vi "F490Y0YIPPPDQXN.vi"() -> ()   [LabVIEW 2014]
uses:
  <vilib>/Utility/error.llb/DialogType.ctl
  <vilib>/addons/Biomedical/Biosignal Measurements/Biosignal Preprocessing/subVIs/bmt_Rate Extractor_peak_valley.ctl
  <vilib>/addons/Biomedical/Biosignal Measurements/Biosignal Preprocessing/Biosignal Rate Extractor (Waveform).vi
  <vilib>/DigilentWF/DigilentWF.lvlib
  <vilib>/addons/Biomedical/NI_BMTK_Measurements.lvlib
panel:
  in  "Acquisition Time":dbl=4.0 caption="Acquisition Time (s) (no change)"
  in  "Sample Rate":dbl=1500.0 caption="Sample Rate (no change)" format="%#_6p"
  in  "On":bool
  in  "UC2":dbl=120.0 caption="Upper Cut-Off"
  in  "LC2":dbl=15.0 caption="Lower Cut-Off"
  out "Smoothing filter":dynamicdata(graph)=[{"t0"=timestamp(0 s since 1904-01-01), "dt"=0.00066667, "Y"=array[6000 elements], "attributes"=variant("NI_ChannelName"=variant(string "Filtered (Filtered)"), "NI_OriginalChannelName"=variant(string "Filtered"))}]
  out "Bandpass filter":dynamicdata(graph)=[{"t0"=timestamp(0 s since 1904-01-01), "dt"=0.00066667, "Y"=array[6000 elements], "attributes"=variant("NI_ChannelName"=variant(string "Filtered (Filtered)"), "NI_OriginalChannelName"=variant(string "Filtered"))}]
  out "Mean Heart Rate":dbl=inf
  in  "HT":dbl(slide)=0.32291666666666663 scale=-0.5..1.5
  in  "LT":dbl(slide)=0.15624999999999997 scale=-0.5..1.5
  out "pulse interval (s)":dbl format="%#.6g"
  out "number of pulses":i32=-1
  out "biosignals":dynamicdata(graph)=[{"t0"=timestamp(0 s since 1904-01-01), "dt"=0.00066667, "Y"=array[6000 elements], "attributes"=variant("NI_ChannelName"=variant(string "Filtered (Filtered)"), "NI_OriginalChannelName"=variant(string "Filtered"))}]
  out "unfiltered":waveform(dbl)(graph)={"t0"=timestamp(3549308991.8308573 s since 1904-01-01), "dt"=0.00066667, "Y"=array[6000 elements]}
  out "Bandpass filter":dynamicdata(graph)=[{"t0"=timestamp(0 s since 1904-01-01), "dt"=0.00066667, "Y"=array[6000 elements], "attributes"=variant("NI_ChannelName"=variant(string "Filtered"))}]
  in  "UC1":dbl=34.0 caption="Upper Cut-Off"
  out "Averaged":waveform(dbl)(graph)={"t0"=timestamp(0 s since 1904-01-01), "dt"=0.00066667, "Y"=array[6000 elements]}
  in  "Samples to Average":i32=10 min=1
  in  "LC1":dbl=1.0 caption="Lower Cut-Off"
  in  "-5V Supply":bool=TRUE
  in  "+5V Supply":bool=TRUE
  in  "Master Enable":bool=TRUE
  in  "V 2":dbl=5.0 caption="Voltage" min=0.5 max=5.0 step=0.1
  in  "V":dbl=-5.0 caption="Voltage" min=-5.0 max=-0.5 step=0.1
  in  "Device Name":string="Analog Discovery 2"
  in  "Stop":bool
  in  "Analog Channel":string="mso/1" caption="Channel"
  # "Heart Rate"
  # "Analog Discovery 2\nPower Supplies"
  # "Analog Discovery MSO Settings"
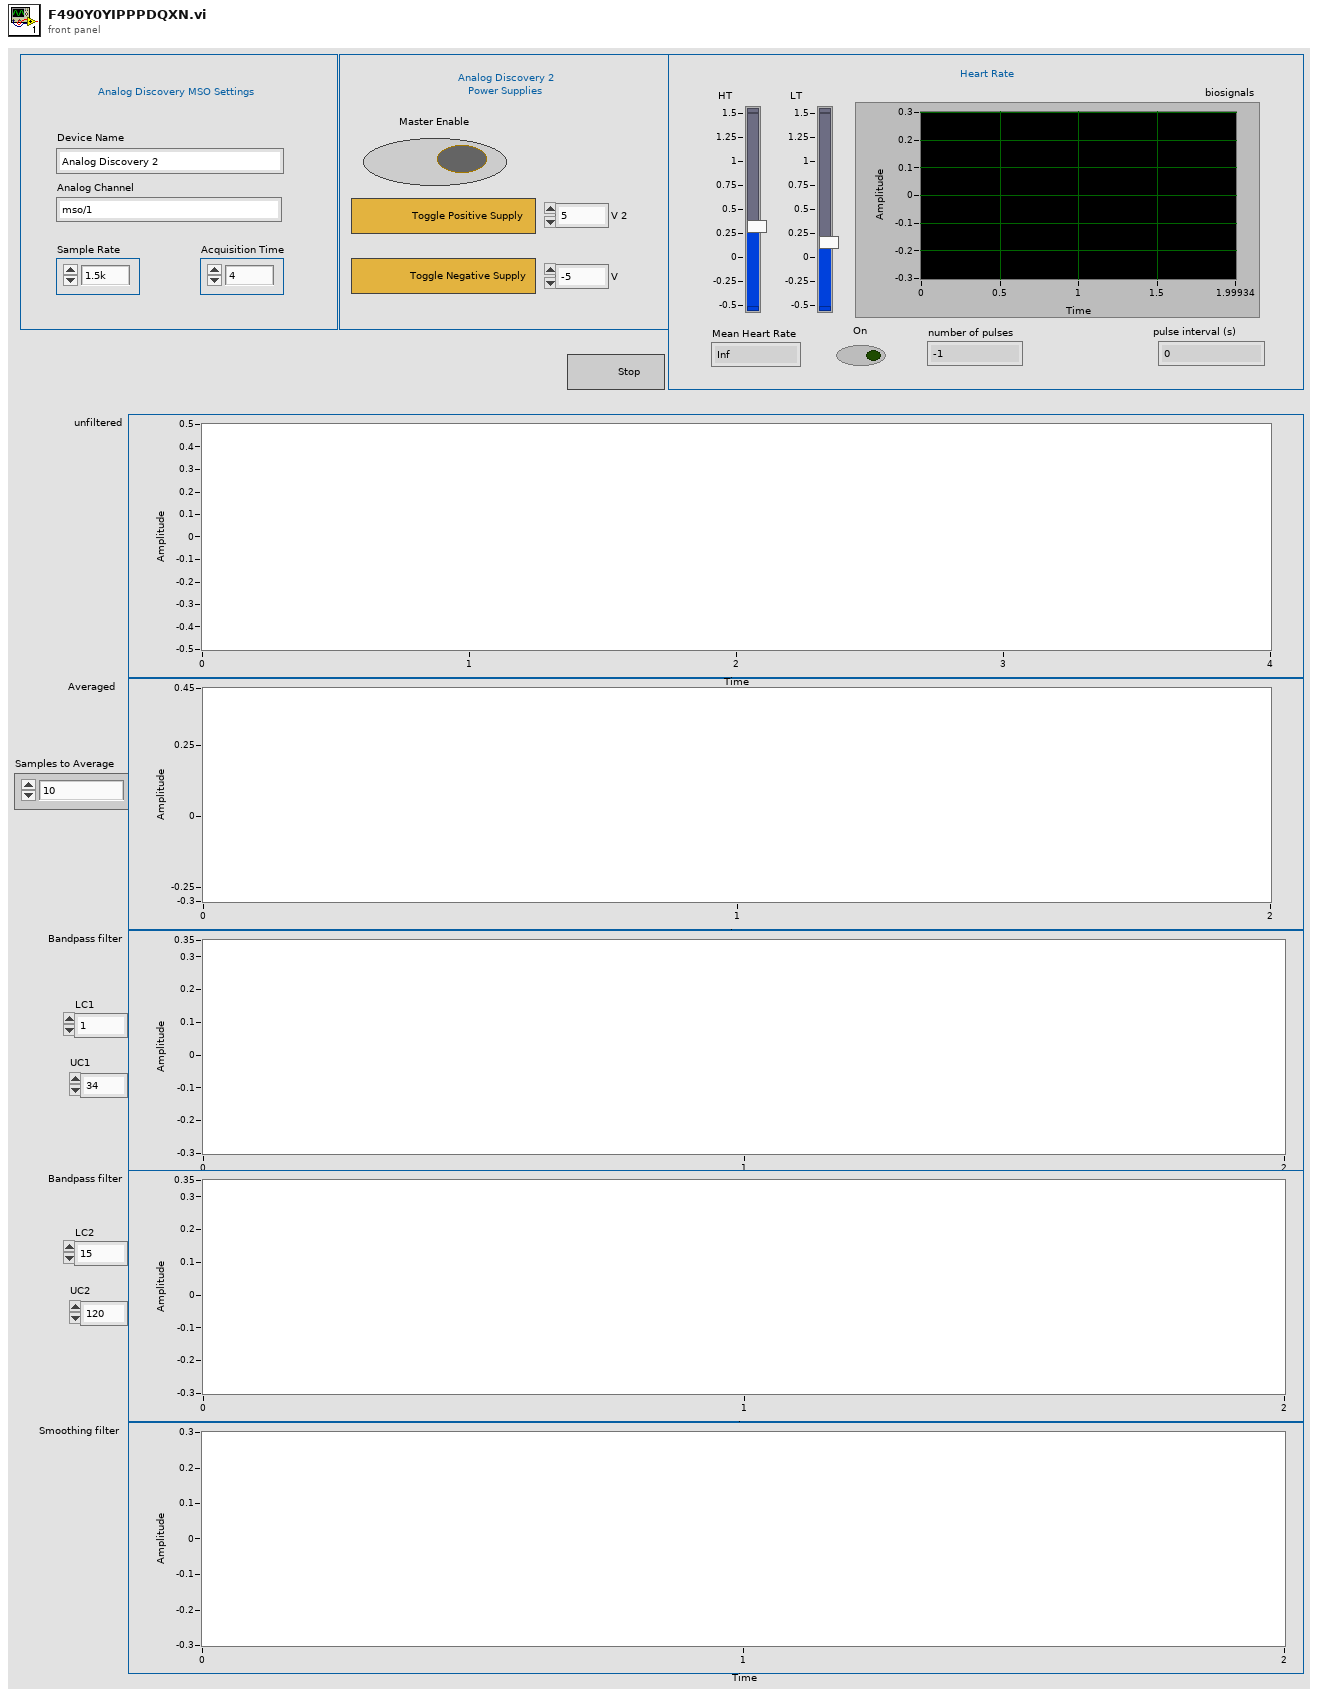
[diagram p1: front panel]
types:
  T1 = typedef "DialogType.ctl" = u16
  T2 = typedef "NI_BMTK_Measurements.lvlib/bmt_Rate Extractor_peak_valley.ctl" = u16
  T3 = typedef "LVCursorListTypeDef.ctl" = cluster{"Name":string, "Color":u32, "Style":u8, "Point Style":u8, "Name Visible":bool, "Allow Drag":bool, "Cursor Mode":u32, "Plot":i32, "Index":i32, "Position":cluster{"X":dbl, "Y":dbl}, "X Scale":u32, "Y Scale":u32, "Watch Plots":i32[], "Watch All Plots":bool, "Plot Area":i32, "Label Offset":cluster{"X":dbl, "Y":dbl}}[]
  T4 = cluster{"Name":string, "Color":u32, "Style":u8, "Point Style":u8, "Name Visible":bool, "Allow Drag":bool, "Cursor Mode":u32, "Plot":i32, "Index":i32, "Position":cluster{"X":dbl, "Y":dbl}, "X Scale":u32, "Y Scale":u32, "Watch Plots":i32[], "Watch All Plots":bool, "Plot Area":i32, "Label Offset":cluster{"X":dbl, "Y":dbl}}
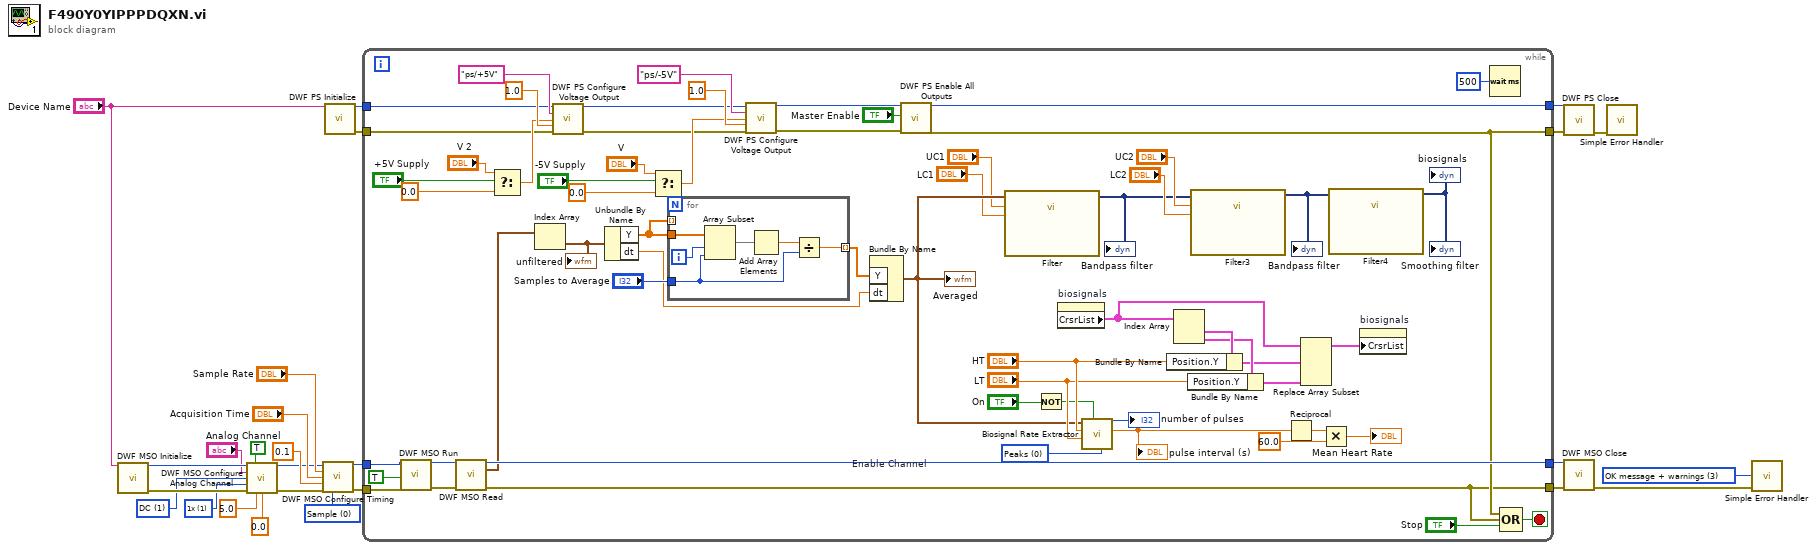
[diagram p0: block diagram]
diagram:
  w6 = 0 items=["Sample", "Peak Detect"] ("Sampling Mode")
  w19 = 1 items=["1x"=1, "10x"=10] ("Probe Attenuation")
  w20 = 1 items=["AC", "DC"] ("Vertical Coupling")
  w25 = TRUE  # Enable Channel
  w26 = T1 3 items=["no dialog", "OK message", "continue or stop message", "OK message + warnings", "continue/stop + warnings"] ("type of dialog (OK msg:1)")
  n1 = call <vilib>:"DWF MSO Initialize.vi"("Device Name"="Device Name") -> ("Instrument Handle Out"=w23:u32, "Error Out"=w24:errorcluster)  [unwired: 13 in]
  n2 = call <vilib>:"DWF MSO Configure Analog Channel.vi"("Instrument Handle In"=w23, "Enable Channel"=w25, "Channel"="Analog Channel", "Vertical Coupling"=w20, "Probe Attenuation"=w19, "Error In"=w24, "Vertical Range"=5.0, "Vertical Offset"=0.0 ("Offset (V)")) -> ("Instrument Handle Out"=w4:u32, "Error Out"=w3:errorcluster)  [unwired: 6 in]
  n3 = call <vilib>:"DWF MSO Configure Timing.vi"("Instrument Handle In"=w4, "Sample Rate"="Sample Rate", "Acquisition Time (s)"="Acquisition Time", "Pretrigger Time (s)"=0.1, "Error In"=w3, "Sampling Mode"=w6) -> ("Instrument Handle Out"=w2:u32, "Error Out"=w1:errorcluster)  [unwired: 8 in]
  n4 = call <vilib>:"DWF PS Initialize.vi"("Device Name"="Device Name") -> ("Instrument Handle Out"=w17:u32, "Error Out"=w16:errorcluster)  [unwired: 13 in]
  n5 = while {
    tunnel: [w86] -> w22
    tunnel: w17 -> [w69]
    tunnel: w16 -> [w68]
    tunnel: [w67] -> w15
    tunnel: [w35] -> w14
    tunnel: [w34] -> w9
    tunnel: w2 -> [w29]
    tunnel: w1 -> [w28]
    stop <- w87 stop-if-true
    w57 = T2 0 items=["Peaks", "Valleys"] ("peaks/valleys")
    n6 = call <vilib>:"DWF MSO Run.vi"("Instrument Handle In"=w29, "Auto Trigger"=TRUE, "Error In"=w28) -> ("Instrument Handle Out"=w65:u32, "Error Out"=w36:errorcluster)  [unwired: 11 in]
    n7 = call <vilib>:"DWF MSO Read.vi"("Instrument Handle In"=w65, "Error In"=w36) -> ("Instrument Handle Out"=w86:u32, "Analog Waveforms"=w60:waveform(dbl)[], "Error Out"=w34:errorcluster)  [unwired: 8 in, 3 out]
    n8 = Select(t="V 2", s="+5V Supply", f=0.0) -> (s? t:f=w76:dbl)
    n9 = Index Array(array=w60) -> (element=w43:waveform(dbl))  [unwired: 1 in]
    "unfiltered" <- w43
    n10 = call <vilib>:"DWF PS Configure Voltage Output.vi"("Instrument Handle In"=w69, "Channel"="ps/+5V", "Voltage Level"=w76, "Current Limit"=1.0, "Error In"=w68) -> ("Instrument Handle Out"=w71:u32, "Error Out"=w72:errorcluster)  [unwired: 9 in]
    n11 = Unbundle By Name(w43) -> ("Y"=w27:dbl[], "dt"=w61:dbl)
    n12 = Select(t="V", s="-5V Supply", f=0.0) -> (s? t:f=w81:dbl)
    n13 = for {
      tunnel: w27 -> [w93]
      tunnel: "Samples to Average" -> [w89]
      tunnel: [w88] -> w62 mode=indexing
      tunnel: w27 -> [_] mode=indexing
      i -> [w92]
      n14 = Array Subset(array=w93, index=w92, length=w89) -> (w91:dbl[])
      n15 = Add Array Elements(numeric array=w91) -> (sum=w90:dbl)
      n16 = Divide(x=w90, y=w89) -> (x/y=w88:dbl)
    }
    n17 = call <vilib>:"DWF PS Configure Voltage Output.vi"("Instrument Handle In"=w71, "Channel"="ps/-5V", "Voltage Level"=w81, "Current Limit"=1.0, "Error In"=w72) -> ("Instrument Handle Out"=w77:u32, "Error Out"=w37:errorcluster)  [unwired: 9 in]
    n18 = Bundle By Name("Y"=w62, "dt"=w61) -> (w45:waveform(dbl))  [unwired: 1 in]
    "Averaged" <- w45
    n19 = call <vilib>:"DWF PS Enable All Outputs.vi"("Instrument Handle In"=w77, "Enable Outputs"="Master Enable", "Error In"=w37) -> ("Instrument Handle Out"=w67:u32, "Error Out"=w35:errorcluster)  [unwired: 11 in]
    n20 = call "Filter"("Lower Cut-Off"="LC1", "Upper Cut-Off"="UC1", "Signal"=w45) -> ("Filtered Signal"=w40:dynamicdata)  [unwired: 7 in, 1 out]
    "Bandpass filter" <- w40
    n21 = Not(x="On") -> (.not. x?=w31:bool)
    n22 = property on="biosignals" class="WFGraph (strict)"() -> ("CrsrList"=w33:T3)  [unwired: 2 in, 2 out]
    n23 = call-poly <vilib>:"Biosignal Rate Extractor.vi"("peaks/valleys"=w57, "initialize? (F)"=w31, "low threshold"="LT", "high threshold"="HT", "biosignal"=w45) -> ("mean cycle time"=w49:dbl, "number of cycles"=→"number of pulses":i32)  [unwired: 4 in, 1 out]
    "pulse interval (s)" <- w49
    n24 = Index Array(array=w33) -> (element #1=w56:T4, element #2=w54:T4)  [unwired: 2 in]
    n25 = Bundle By Name(cluster=w56, "Position.Y"="HT") -> (w52:T4)
    n26 = Bundle By Name(cluster=w54, "Position.Y"="LT") -> (w51:T4)
    n27 = call "Filter3"("Lower Cut-Off"="LC2", "Upper Cut-Off"="UC2", "Signal"=w40) -> ("Filtered Signal"=w44:dynamicdata)  [unwired: 7 in, 1 out]
    "Bandpass filter" <- w44
    n28 = Reciprocal(x=w49) -> (1/x=w48:dbl)
    n29 = Replace Array Subset(array=w33, new element #1=w52, new element #2=w51) -> (w50:T3)  [unwired: 2 in]
    n30 = Multiply(x=w48, y=60.0) -> (x*y=→"Mean Heart Rate":dbl)
    n31 = call "Filter4"("Signal"=w44) -> ("Filtered Signal"=→"biosignals" →"Smoothing filter":dynamicdata)  [unwired: 9 in, 1 out]
    n32 = property on="biosignals" class="WFGraph (strict)"("CrsrList"=w50) -> ()  [unwired: 2 in, 2 out]
    n33 = Wait (ms)(milliseconds to wait=u32 500) -> ()  [unwired: 1 out]
    n34 = Compound Arithmetic op=OR(w35, w34, "Stop") -> (w87:bool)
  }
  n35 = call <vilib>:"DWF PS Close.vi"("Instrument Handle In"=w15, "Error In"=w14) -> ("Error Out"=w18:errorcluster)  [unwired: 13 in]
  n36 = call <vilib>:"DWF MSO Close.vi"("Instrument Handle In"=w22, "Error In"=w9) -> ("Error Out"=w12:errorcluster)  [unwired: 13 in]
  n37 = call <vilib>:"Simple Error Handler.vi"("error in (no error)"=w18) -> ()  [unwired: 4 in, 5 out]
  n38 = call <vilib>:"Simple Error Handler.vi"("type of dialog (OK msg:1)"=w26, "error in (no error)"=w12) -> ()  [unwired: 3 in, 5 out]
